vi "colourByStage.vi"(8 "error in (no error)":errorcluster, 11 "ScriptEditorV2 in":refnum<class "ScriptEditorV2.lvclass">) -> (0 "error out":errorcluster, 3 "ScriptEditorV2 out":refnum<class "ScriptEditorV2.lvclass">)   [LabVIEW 2011, in "Views.lvlib" / "ScriptEditor.lvlib" / "ScriptEditorV2.lvclass"]
uses:
  ScriptEditorV2.lvclass
  ScriptEditorV2.lvclass/ScriptEditorV2.ctl
  Tools/DatabaseHelpers/DbConnection/DeviceDataBase/deviceDataBase.lvclass
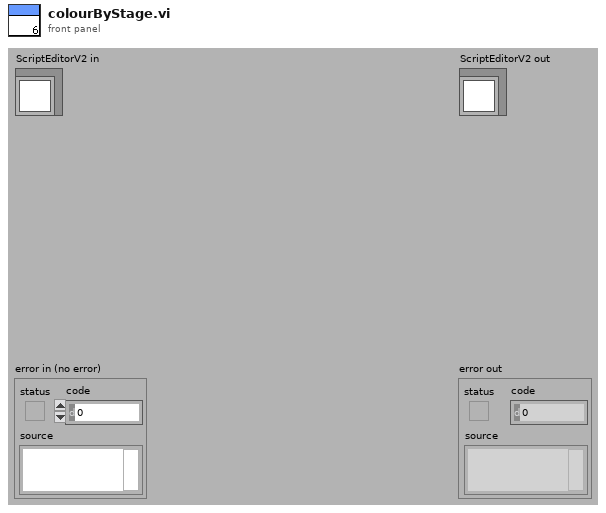
[diagram p1: front panel]
types:
  T1 = typedef "LVRowAndColumnUnsignedTypeDef.ctl" = cluster{"Row":u32, "Column":u32}
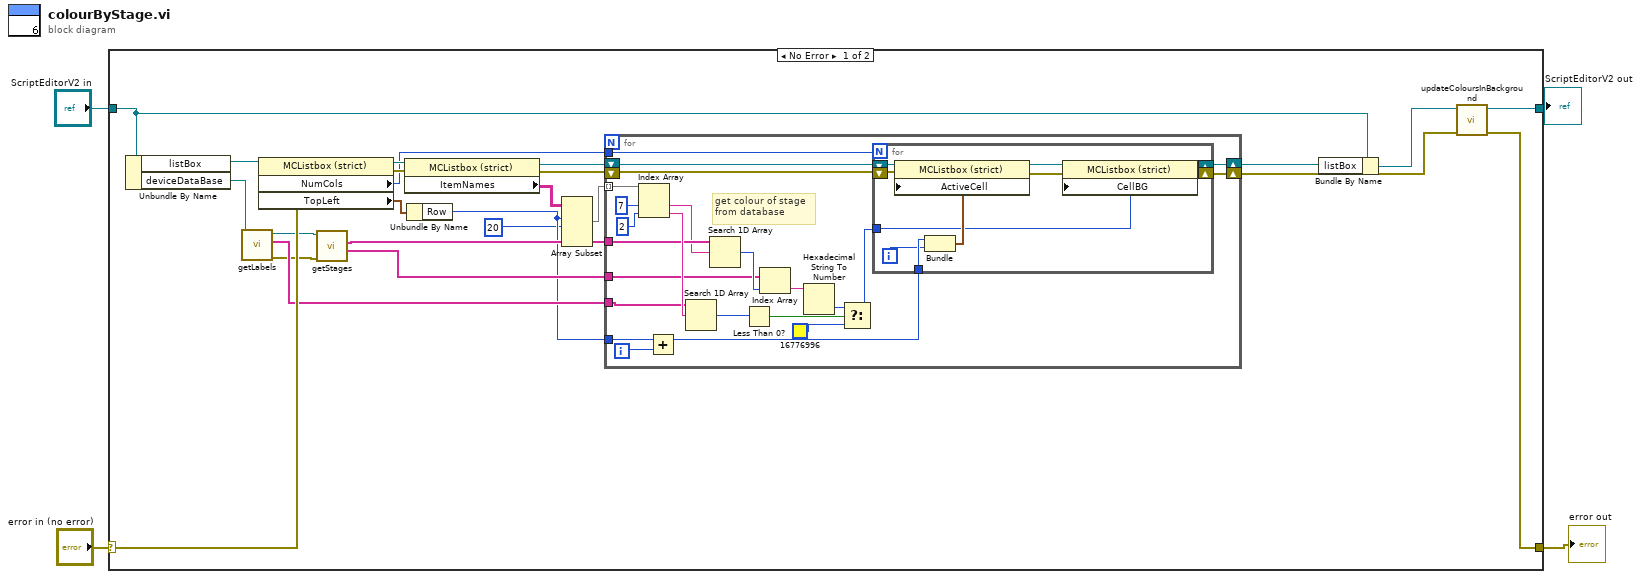
[diagram p0: block diagram]
diagram:
  n1 = case shown="No Error" "error in (no error)" {
    selector: "error in (no error)" -> [w25 w63]
    tunnel: [w8 w63] -> w3
    tunnel: [w10 w62] -> w1
    tunnel: "ScriptEditorV2 in" -> [w22 w62]
    frame No Error {
      n2 = Unbundle By Name(w22) -> ("listBox"=w24:refnum<vi>, "deviceDataBase"=w19:refnum<class "deviceDataBase.lvclass">)
      n3 = call "getLabels.vi"("deviceDataBase in"=w19) -> ("error out"=w16:errorcluster, "labels"=w18:string[], "deviceDataBase out"=w17:refnum<class "deviceDataBase.lvclass">)  [unwired: 8 in]
      n4 = property class="MCListbox (strict)"(reference=w24, error in=w25) -> (reference out=w27:refnum<vi>, error out=w26:errorcluster, "NumCols"=w23:u32, "TopLeft"=w7:T1)
      n5 = call "getStages.vi"("error in (no error)"=w16, "deviceDataBase in"=w17) -> ("colours"=w14:string[], "stages"=w15:string[])  [unwired: 6 in, 2 out]
      n6 = property class="MCListbox (strict)"(reference=w27, error in=w26) -> (reference out=w28:refnum<vi>, error out=w20:errorcluster, "ItemNames"=w13:string[][])
      n7 = Unbundle By Name(w7) -> ("Row"=w6:u32)
      n8 = Array Subset(array=w13, index (row)=w6, length (row)=20) -> (w12:string[][])  [unwired: 2 in]
      n9 = for {
        tunnel: w12 -> [w51] mode=indexing
        tunnel: w23 -> [w48]
        shift-right: [w47] -> w21
        shift-left: w28 -> [w49]
        shift-right: [w45] -> w9
        shift-left: w20 -> [w46]
        tunnel: w18 -> [w42]
        tunnel: w15 -> [w37]
        tunnel: w14 -> [w35]
        tunnel: w6 -> [w31]
        i -> [w29]
        # "get colour of stage\nfrom database"
        n10 = Index Array(array=w51, index #1=7, index #2=2) -> (element #1=w34:string, element #2=w43:string)
        n11 = Add(x=w31, y=w29) -> (x+y=w30:u32)
        n12 = Search 1D Array(1D array=w42, element=w43) -> (index of element=w38:i32)  [unwired: 1 in]
        n13 = Search 1D Array(1D array=w37, element=w34) -> (index of element=w36:i32)  [unwired: 1 in]
        n14 = Less Than 0?(x=w38) -> (x < 0?=w41:bool)
        n15 = Index Array(array=w35, index=w36) -> (element=w32:string)
        n16 = Hexadecimal String To Number(string=w32) -> (number=w33:u32)  [unwired: 2 in, 1 out]
        n17 = Select(t=w33, s=w41, f=u32 16776996) -> (s? t:f=w40:u32)
        n18 = for {
          N: w48 -> [_]
          tunnel: w30 -> [w53]
          shift-right: [w57] -> w47
          shift-left: w49 -> [w60]
          shift-right: [w55] -> w45
          shift-left: w46 -> [w56]
          tunnel: w40 -> [w54]
          i -> [w52]
          n19 = Bundle(w53, w52) -> (w58:cluster{u32, i32})  [unwired: 1 in]
          n20 = property class="MCListbox (strict)"(reference=w60, error in=w56, "ActiveCell"=w58) -> (reference out=w61:refnum<vi>, error out=w59:errorcluster)
          n21 = property class="MCListbox (strict)"(reference=w61, error in=w59, "CellBG"=w54) -> (reference out=w57:refnum<vi>, error out=w55:errorcluster)
        }
      }
      n22 = Bundle By Name(cluster=w22, "listBox"=w21) -> (w11:refnum<class "ScriptEditorV2.lvclass">)
      n23 = call "updateColoursInBackground.vi"("error in (no error)"=w9, "ScriptEditorV2 in"=w11) -> ("error out"=w8:errorcluster, "ScriptEditorV2 out"=w10:refnum<class "ScriptEditorV2.lvclass">)  [unwired: 8 in]
    }
    frame Error {
    }
  }
  "error out" <- w3
  "ScriptEditorV2 out" <- w1
